vi "Rapid Read_Alazar_Done - ATS-SDK.vi"(0 "Handle":u32, 1 "Motion Settings":T1={"No Motion?"=FALSE, "Motion System"=enum."NI 735x", "Motion Bd ID"=1, "Motion Profile"="SMAC1", "# Axis"=1, "Reverse Z axis?"=TRUE, "SMAC Axis"=0, "scan pair"=enum."y-(x) scan", "RT fps"=6.0, "Steps per mm"=[1000, 1000, 1000, 1000], "Motor Parameters"={"velocity ct/s"=[10000.0, 10000.0, 10000.0, 50000.0], "accel ct/s^2"=[50000.0, 50000.0, 50000.0, 200000.0]}, "One Way Scan"=FALSE, "Reverse One Way Scan"=FALSE, "Global Position (mm)"=[], "Plane"=0, "Distance between\nscan lines (um)"=0.0, "Distance between\nscan planes (um)"=0.0, "number of scan planes"=1, "Total steps in line"=0, "Xtra plane\ndistance  (um)"=100, "Xtra planes "=1, "Add Axis"=FALSE, "overshoot cts"=200, "BKPT Shift"=0, "Scan Start Time (ms)"=0, "ESP VISA"="GPIB::1::INSTR", "3rd Axis"=1, "GL Ref Out"=refnum, "Galil Address"=""} {"3rd Axis" items=["x", "y", "z", "w"]; "Xtra planes" min=1; "Xtra plane\ndistance  (um)" min=0; "Distance between\nscan planes (um)" format="%.2f"; "Distance between\nscan lines (um)" format="%.2f"; "SMAC Axis" items=["None"=0, "Axis 1"=1, "Axis 2"=2, "Axis 3"=3, "Axis 4"=4, "Axis 5"=5, "Axis 6"=6, "Axis 7"=7, "Axis 8"=8, "Vector Space 1"=17, "Vector Space 2"=18, "Vector Space 3"=19, "Vector Space 4"=20]; "Motion Bd ID" min=1 max=32 step=1}, 11 "error out":errorcluster, 14 "Pause?":bool) -> (4 "Handle Out":u32, 6 "Reverse?":bool, 15 "error out":errorcluster)   [LabVIEW 2022 SP3]
uses:
  Motion Controllers/NI_controller/-NI_MotionRoutines/MotionParameters.ctl
  Motion Controllers/NI_controller/-NI_MotionRoutines/MotionSys.ctl
  Motion Controllers/-MotionRoutines/ScanAxis.ctl
  Motion Controllers/-MotionRoutines/3rdAxis.ctl
  <vilib>/Platform/TimedLoop/XDataNode/timing_clust.ctl
  <vilib>/Platform/TimedLoop/XDataNode/nitl_modes.ctl
  <vilib>/Platform/TimedLoop/XDataNode/wakeup.ctl
  Motion Controllers/Galil/Command Menu.ctl
  <vilib>/Platform/TimedLoop/XDataNode/XDataNode.xnode
  <vilib>/Platform/TimedLoop/XDataNode/XDNodeRunTimeDep.lvlib
panel:
  # "1-D and 2-D B scan settings"
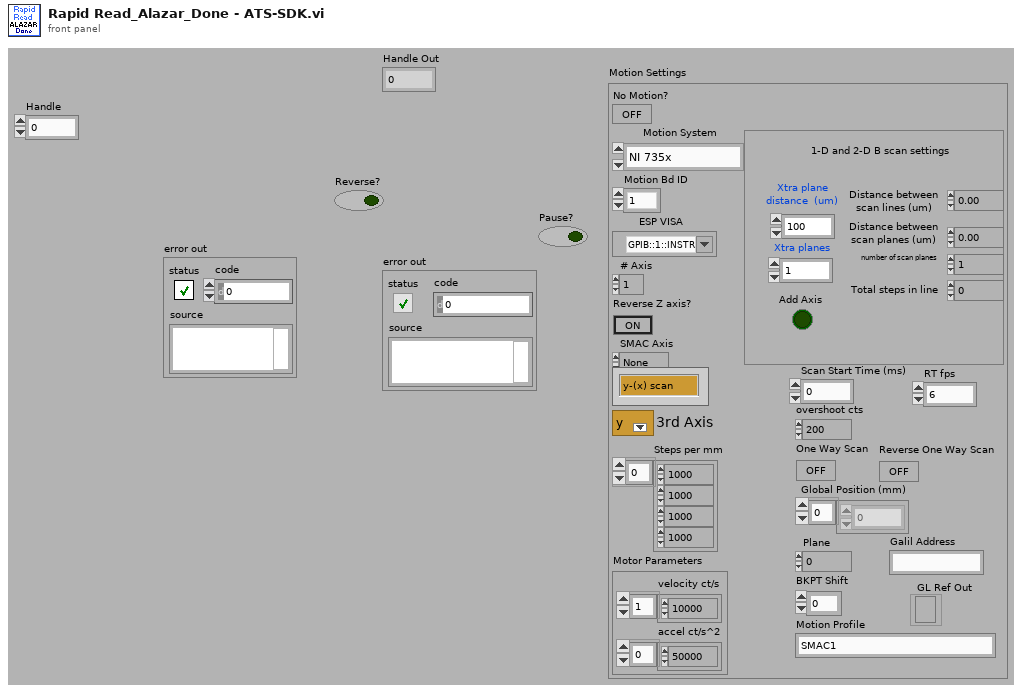
[diagram p1: front panel]
types:
  T1 = typedef "MotionParameters.ctl" = cluster{"No Motion?":bool, "Motion System":T2, "Motion Bd ID":u8, "Motion Profile":string, "# Axis":i8, "Reverse Z axis?":bool, "SMAC Axis":u16, "scan pair":T3, "RT fps":sgl, "Steps per mm":i32[], "Motor Parameters":cluster{"velocity ct/s":dbl[], "accel ct/s^2":dbl[]}, "One Way Scan":bool, "Reverse One Way Scan":bool, "Global Position (mm)":dbl[], "Plane":i32, "Distance between\nscan lines (um)":sgl, "Distance between\nscan planes (um)":sgl, "number of scan planes":i32, "Total steps in line":i32, "Xtra plane\ndistance  (um)":i32, "Xtra planes ":i32, "Add Axis":bool, "overshoot cts":i32, "BKPT Shift":i32, "Scan Start Time (ms)":u32, "ESP VISA":refnum<visa-resource-name>, "3rd Axis":T4, "GL Ref Out":refnum<k7>, "Galil Address":string}
  T2 = typedef "MotionSys.ctl" = enum16{"MM3000", "NI 735x", "Newport ESP", "No Motion Card", "Galil"}
  T3 = typedef "ScanAxis.ctl" = enum16{"y-(x) scan", "x-(y) scan", "z-(x) scan", "z-(y) scan", "y-(z) scan", "x-(z) scan", "w-(x) scan", "w-(y) scan", "w-(z) scan", "x-(w) scan", "y-(w) scan", "z-(w) scan"}
  T4 = typedef "3rdAxis.ctl" = u16
  T5 = typedef "Command Menu.ctl" = enum16{"CommandPassThrough", "Abort Motion", "Define Pos", "Velocity", "Acceleration", "Deceleration", "Position Rel", "Postion Abs", "Begin Move", "After Move", "Home", "KI", "KD", "KP", "IL", "Config I/O", "Set Bit", "Clear Bit", "Motor Off", "Moto On", "Status", "Execute", "Halt Execute", "HX Status", "Tell Velocity", "Check Motion", "BreakPoint", "Tell Position", "Current Code Line", "Tell Switches", "OC Force On", "OC Off", "Pos Soft Limit", "Rev Soft Limit"}
  T6 = typedef "XDNodeRunTimeDep.lvlib/timing_clust.ctl" = cluster{"Expected End [f-1]":u64, "Actual End [f-1]":u64, "Finished Late? [f-1]":bool, "Expected End [i-1]":u64, "Actual End [i-1]":u64, "Finished Late? [i-1]":bool, "Expected Start [i]":u64, "Actual Start [i]":u64, "Expected Start [f]":u64, "Actual Start [f]":u64, "Source Name":string, "Structure Name":string, "Period":i64, "Deadline":i64, "Offset":i64, "Start":i64, "Priority":i32, "Timeout":i32, "Mode":T7, "Wakeup Reason":T8, "Error":errorcluster, "Source Type":string, "Secondary Source Type":string, "Global End Time":u64, "Global Start Time":u64, "Frame Duration":u64, "Iteration Duration":u64, "Assigned CPU":i32, "I/O Scan Engine Mode":u32}
  T7 = typedef "XDNodeRunTimeDep.lvlib/nitl_modes.ctl" = enum32{"No Change", "Process missed periods, maintain original phase", "Discard missed periods, maintain original phase", "Process missed periods, ignore original phase", "Discard missed periods, ignore original phase"}
  T8 = typedef "XDNodeRunTimeDep.lvlib/wakeup.ctl" = enum32{"Normal", "Aborted", "Asynchronous wakeup", "Timing source error", "Timed loop error", "Timeout"}
  T9 = typedef "Var" = u8
  T10 = typedef "Bd Id Out" = u8
  T11 = cluster{"Run/Stop":bool, "Profile Complete":bool, "Motor Off ":bool, "Following Error":bool, "Limit Switch":bool, "Home Switch":bool, "SW Limit Switch":bool, "Watchdog":bool, "Velocity Threshold":bool, "Position Brkpt":bool, "Home Found":bool, "Index Found":bool, "High Speed Capture":bool, "Reverse Direction":bool, "Blend Complete":bool, "Move Complete":bool}
  T12 = typedef "GL Axis Control.ctl" = u16
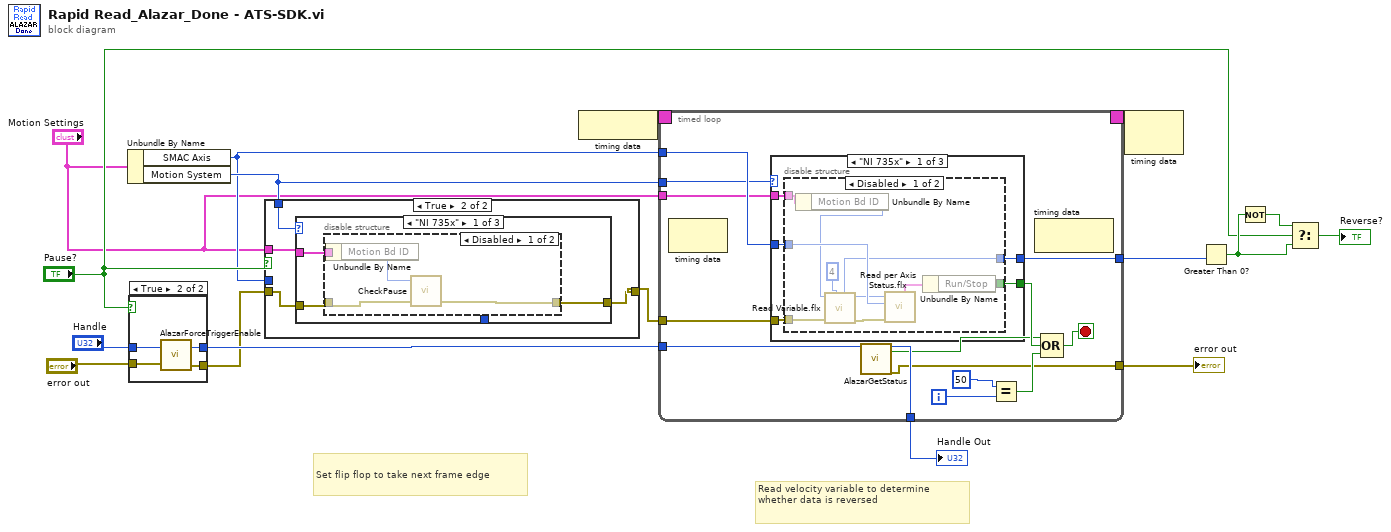
[diagram p0: block diagram]
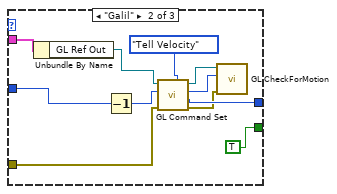
[diagram p4: hidden frame]
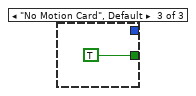
[diagram p5: hidden frame]
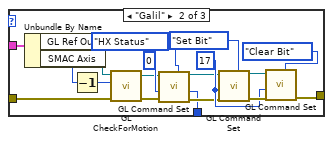
[diagram p8: hidden frame]
diagram:
  # "Set flip flop to take next frame edge"
  # "Read velocity variable to determine whether data is reversed"
  n1 = Unbundle By Name("Motion Settings") -> ("SMAC Axis"=w2:u16, "Motion System"=w3:T2)
  n2 = case shown="True" "Pause?" {
    tunnel: [w19 w23] -> w14
    tunnel: "Handle" -> [w19 w22]
    tunnel: "error out" -> [w18 w21]
    tunnel: [w18 w20] -> w8
    frame False {
    }
    frame True {
      n3 = call "AlazarForceTriggerEnable.vi"("Handle"=w22, "error in (no error)"=w21) -> ("Handle"=w23:u64, "error out"=w20:errorcluster)  [unwired: 1 out]
    }
  }
  n4 = case shown="True" "Pause?" {
    tunnel: w8 -> [w24 w27]
    tunnel: w3 -> [_ w25]
    tunnel: [w24 w28] -> w4
    tunnel: w2 -> [_ _]
    tunnel: "Motion Settings" -> [_ w26]
    frame False {
    }
    frame True {
      n5 = case shown="\"NI 735x\"" w25 {
        tunnel: [w31 w49 w54] -> w28
        tunnel: w27 -> [w30 w52 w54]
        tunnel: w26 -> [w29 w45 _]
        tunnel: [_ w36 _] -> _
        frame "NI 735x" {
          n6 = disable-structure shown="Disabled" {
            disable-tunnel: [w35 _] -> w31
            disable-tunnel: w30 -> [w34 _]
            disable-tunnel: w29 -> [w33 _]
            frame Disabled {
              n7 = Unbundle By Name(w33) -> ("Motion Bd ID"=w32:u8)
              n8 = call "CheckPause.vi"("error in"=w34, "Motion Board ID"=w32) -> ("error out"=w35:errorcluster)  [unwired: 3 in]
            }
            frame Enabled {
            }
          }
        }
        frame "Galil" {
          w46 = 17 ("Value")
          n9 = Unbundle By Name(w45) -> ("GL Ref Out"=w44:refnum<k7>, "SMAC Axis"=w43:u16)
          n10 = Decrement(x=w43) -> (x-1=w53:u16)
          n11 = call "GL CheckForMotion.vi"("error in"=w52, "Axis"=w53, "Refnum in"=w44) -> ("error out"=w40:errorcluster, "Refnum out"=w37:refnum<k7>)  [unwired: 6 in, 1 out]
          n12 = call "GL Command Set.vi"("Command"=Command_Menu."HX Status", "error in (no error)"=w40, "Value"=0, "Galil.IGalil"=w37) -> ("error out"=w39:errorcluster, "Response#"=w36:i32, "ref out"=w38:refnum<k7>)  [unwired: 3 in, 2 out]
          n13 = call "GL Command Set.vi"("Command"=Command_Menu."Set Bit", "error in (no error)"=w39, "Value"=w46, "Galil.IGalil"=w38) -> ("error out"=w50:errorcluster, "ref out"=w47:refnum<k7>)  [unwired: 3 in, 3 out]
          n14 = call "GL Command Set.vi"("Command"=Command_Menu."Clear Bit", "error in (no error)"=w50, "Value"=w46, "Galil.IGalil"=w47) -> ("error out"=w49:errorcluster)  [unwired: 3 in, 4 out]
        }
        frame "No Motion Card", Default {
        }
      }
    }
  }
  n15 = node-c288() -> (w16:T6)
  n16 = timed-loop {
    timing: w16 -> [_]
    timing-out: [_] -> w15
    tunnel: w14 -> [w61]
    tunnel: w2 -> [w64]
    tunnel: w3 -> [w63]
    tunnel: [w60] -> w10
    tunnel: [w58] -> w6
    tunnel: w4 -> [w57]
    tunnel: [w56] -> w7
    tunnel: "Motion Settings" -> [w55]
    i -> [w68]
    stop <- w67 stop-if-true
    n17 = node-c288() -> ()  [unwired: 1 in, 1 out]
    n18 = case shown="\"NI 735x\"" w63 {
      tunnel: w64 -> [w73 w93 _]
      tunnel: [w72 TRUE ("Run/Stop") TRUE ("Run/Stop")] -> w62
      tunnel: w57 -> [w71 w86 _]
      tunnel: [w70 w91 _] -> w56
      tunnel: w55 -> [w69 w85 _]
      frame "NI 735x" {
        n19 = disable-structure shown="Disabled" {
          disable-tunnel: w73 -> [w83 _]
          disable-tunnel: [w81 _] -> w72
          disable-tunnel: w71 -> [w80 _]
          disable-tunnel: [w77 _] -> w70
          disable-tunnel: w69 -> [w75 _]
          frame Disabled {
            n20 = Unbundle By Name(w75) -> ("Motion Bd ID"=w74:u8)
            n21 = call <vilib>:"Read Variable.flx"("Var"=T9 4, "error in (no error)"=w80, "Board ID"=w74) -> ("error out"=w79:errorcluster, "Bd ID Out"=w76:T10, "Output"=w77:i32)  [unwired: 1 in, 3 out]
            n22 = call <vilib>:"Read per Axis Status.flx"("error in (no error)"=w79, "Axis"=w83, "Board ID"=w76) -> ("Per Axis H/W Status"=w82:T11)  [unwired: 3 in, 3 out]
            n23 = Unbundle By Name(w82) -> ("Run/Stop"=w81:bool)
          }
          frame Enabled {
          }
        }
      }
      frame "Galil" {
        n24 = Unbundle By Name(w85) -> ("GL Ref Out"=w84:refnum<k7>)
        n25 = Decrement(x=w93) -> (x-1=w90:u16)
        n26 = call "GL Command Set.vi"("Command"=Command_Menu."Tell Velocity", "error in (no error)"=w86, "Axis"=w90, "Galil.IGalil"=w84) -> ("error out"=w88:errorcluster, "Response#"=w91:i32, "Axis Out"=w89:T12, "ref out"=w92:refnum<k7>)  [unwired: 3 in, 1 out]
        n27 = call "GL CheckForMotion.vi"("error in"=w88, "Axis"=w89, "Refnum in"=w92) -> ()  [unwired: 6 in, 3 out]
      }
      frame "No Motion Card", Default {
      }
    }
    n28 = call "AlazarGetStatus.vi"("Handle"=w61) -> ("Handle"=w60:u64, "Trig. Timeout"=w59:bool, "error out"=w58:errorcluster)  [unwired: 13 in, 3 out]
    n29 = Equal?(x=50, y=w68) -> (x = y?=w65:bool)
    n30 = node-c288() -> ()  [unwired: 1 in, 1 out]
    n31 = Compound Arithmetic op=OR(w59, w62, w65) -> (w67:bool)
  }
  "error out" <- w6
  "Handle Out" <- w10
  n32 = node-c288(w15) -> ()  [unwired: 1 out]
  n33 = Greater Than 0?(x=w7) -> (x > 0?=w13:bool)
  n34 = Not(x=w13) -> (.not. x?=w12:bool)
  n35 = Select(t=w12, s="Pause?", f=w13) -> (s? t:f=→"Reverse?":bool)
